vi "Dispense test.vi"() -> ()   [LabVIEW 2019]
uses:
  Classes/Controller/Dispenser/Dispenser.lvclass
  Classes/Controller/Controller.lvclass
panel:
  out "error out":errorcluster
  in  "error in (no error)":errorcluster
  in  "Pressure":i16=20
  in  "Dispense":bool
  in  "stop":bool
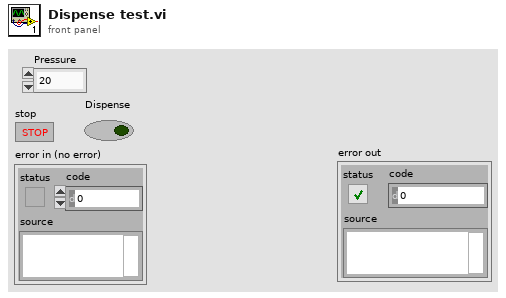
[diagram p1: front panel]
types:
  T1 = typedef "Controller.lvclass/Controllers.ctl" = cluster{"I-O.lvclass":refnum<class "I-O.lvclass">, "Dispenser.lvclass":refnum<class "Dispenser.lvclass">, "Gantry":refnum<k24>}
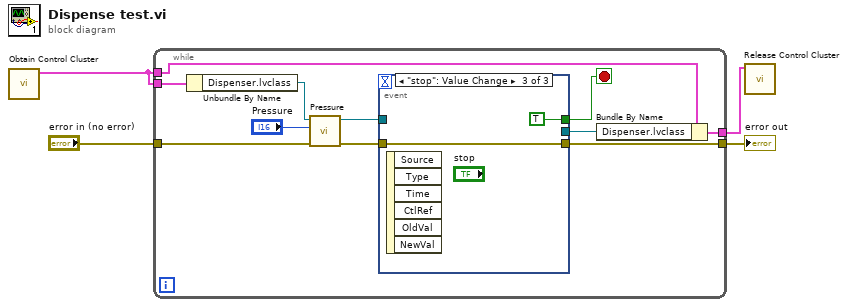
[diagram p0: block diagram]
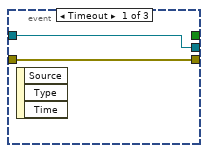
[diagram p2: hidden frame]
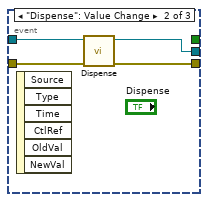
[diagram p3: hidden frame]
diagram:
  n1 = call "Obtain Control Cluster.vi"() -> ("Control Out"=w3:T1)  [unwired: 11 in]
  n2 = while {
    tunnel: w3 -> [w15]
    tunnel: "error in (no error)" -> [w12]
    tunnel: w3 -> [w9]
    tunnel: [w8] -> w2
    tunnel: [w6] -> w1
    stop <- w5 stop-if-true
    n3 = Unbundle By Name(w15) -> ("Dispenser.lvclass"=w14:refnum<class "Dispenser.lvclass">)
    n4 = call-dynamic "Pressure.vi"("error in (no error)"=w12, "Pressure"="Pressure", "Dispenser in"=w14) -> ("error out"=w7:errorcluster, "Dispenser out"=w11:refnum<class "Dispenser.lvclass">)  [unwired: 7 in]
    n5 = event shown="[2] \"stop\": Value Change" {
      selector: _ -> [_ _ _]
      dyn-events: _ -> [_ _ _]
      timeout: _ -> [_ _ _]
      tunnel: w11 -> [w17 w21 _]
      tunnel: [w17 w20 _] -> w10
      tunnel: w7 -> [w16 w19 w23]
      tunnel: [w16 w18 w23] -> w6
      tunnel: [_ _ TRUE] -> w5
      event Timeout {
        n6 = event-data() -> ()  [unwired: 1 in, 3 out]
      }
      event "Dispense": Value Change {
        n7 = event-data() -> ()  [unwired: 1 in, 6 out]
        n8 = call-dynamic "Dispense.vi"("error in (no error)"=w19, "Dispenser in"=w21) -> ("error out"=w18:errorcluster, "Dispenser out"=w20:refnum<class "Dispenser.lvclass">)  [unwired: 8 in]
      }
      event "stop": Value Change {
        n9 = event-data() -> ()  [unwired: 1 in, 6 out]
      }
    }
    n10 = Bundle By Name(cluster=w9, "Dispenser.lvclass"=w10) -> (w8:T1)
  }
  "error out" <- w1
  n11 = call "Release Control Cluster.vi"("output cluster"=w2) -> ()  [unwired: 11 in]
